vi "smartAddition.vi"(10 "x":dbl, 11 "old x":dbl) -> (2 "y":dbl)   [LabVIEW 2020]
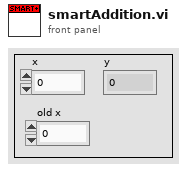
[diagram p1: front panel]
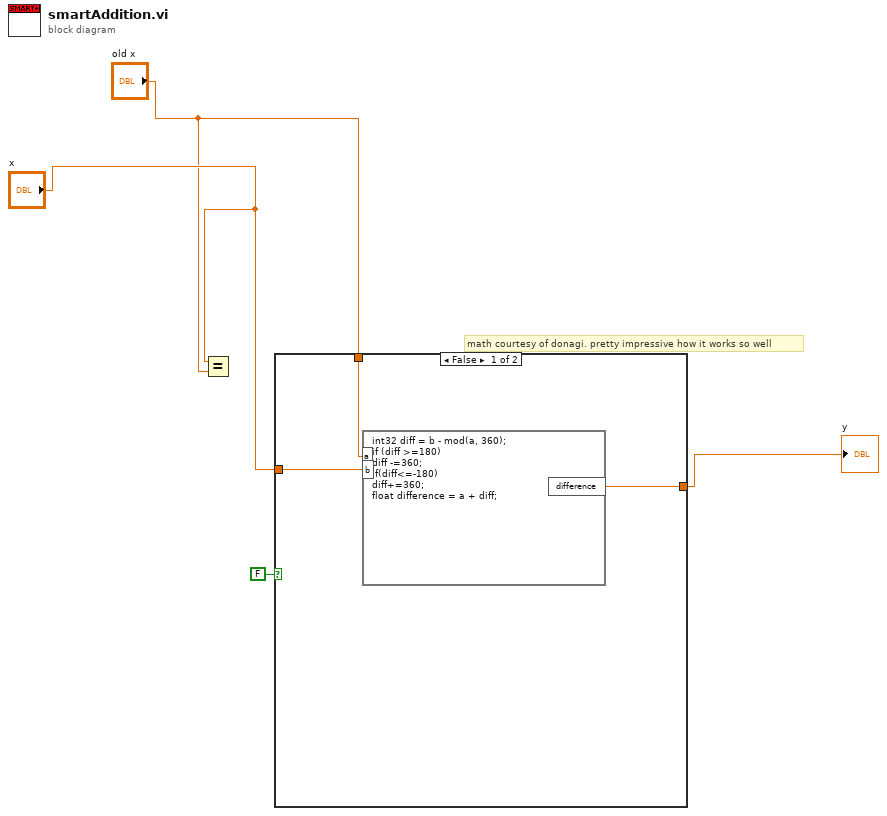
[diagram p0: block diagram]
diagram:
  # "math courtesy of donagi. pretty impressive how it works so well"
  n1 = Equal?(x="x", y="old x") -> ()  [unwired: 1 out]
  n2 = case shown="False" FALSE {
    tunnel: "old x" -> [w7 _]
    tunnel: "x" -> [w6 w8]
    tunnel: [w5 w8] -> w3
    frame False {
      n3 = formula code="int32 diff = b - mod(a, 360);\nif (diff >=180)\ndiff -=360;\nif(diff<=-180)\ndiff+=360;\nfloat difference = a + diff;"("a"=w7, "b"=w6) -> ("difference"=w5:dbl)
    }
    frame True {
    }
  }
  "y" <- w3
